vi "BentStyle_GetObjectStatus.vi"(0 "reference in":refnum<class "BentStyle.lvclass">, 5 "error in (no error)":errorcluster) -> (14 "reference out":refnum<class "BentStyle.lvclass">, 16 "Object name":string, 19 "error out":errorcluster)   [LabVIEW 2012, in "BentStyle.lvclass"]
doc: "Returns the object status and also information about all the objects in the class.\n\n[GOOP 2.0.15]"
uses:
  <resource>/Framework/Providers/Open_GDS/UML/BentStyle_class/BentStyle.lvclass
  <resource>/Framework/Providers/Open_GDS/UML/BentStyle_class/BentStyle.lvclass/BentStyle.ctl
panel:
  in  "DebuggerInput":string
  out "DebuggerOutput":string
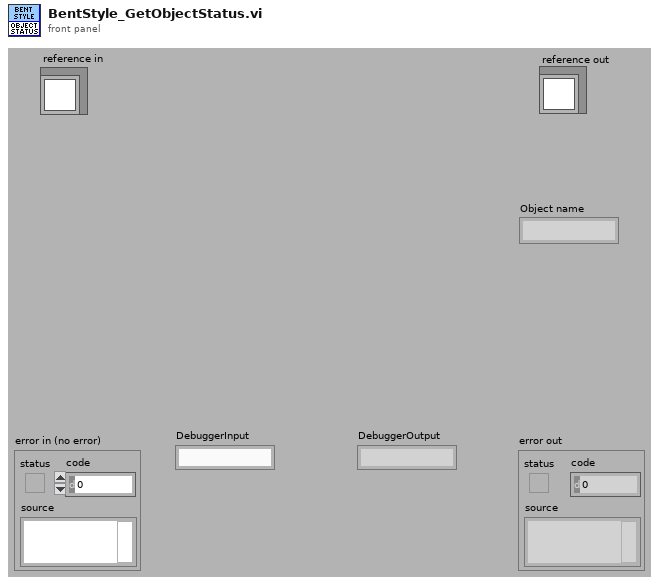
[diagram p1: front panel]
types:
  T1 = typedef "BentStyle.lvclass/BentStyleType.ctl" = enum16{"STRAIGHT", "HV", "VH", "HVH", "VHV", "ARC"}
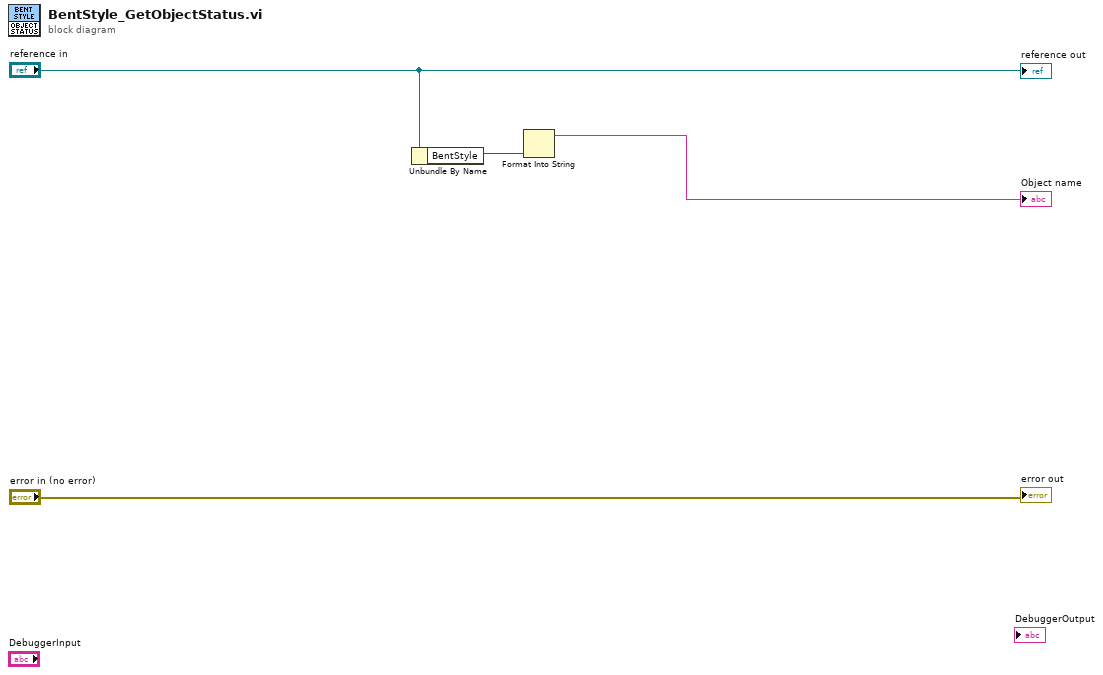
[diagram p0: block diagram]
diagram:
  n1 = Unbundle By Name("reference in") -> ("BentStyle"=w2:T1)
  n2 = Format Into String(w2) -> (resulting string=→"Object name":string)  [unwired: 3 in, 1 out]
  "error out" <- "error in (no error)"
  "reference out" <- "reference in"
